vi "1CLABVIEW.vi"() -> ()   [LabVIEW 2013]
panel:
  out "CARRY":bool
  out "SUM":bool
  out "CARRY":bool
  out "SUM":bool
  in  "Cin":bool
  in  "B":bool
  in  "A":bool
  in  "B":bool
  in  "A":bool
  # "1(c).HALF ADDER and  FULL ADDER"
  # "O.SRINIVAS\n23A91A04H6"
  # "Half adder"
  # "Full adder"
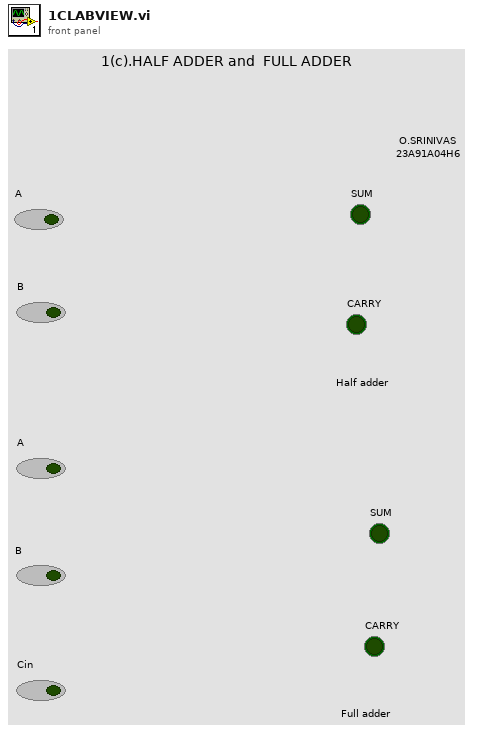
[diagram p1: front panel]
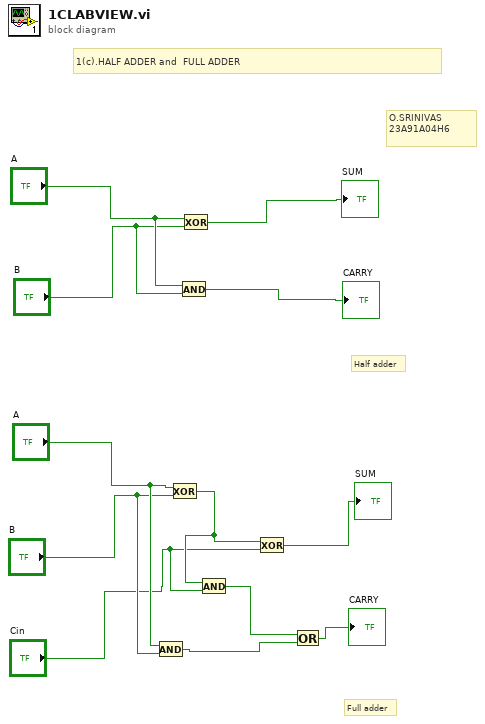
[diagram p0: block diagram]
diagram:
  # "Full adder"
  # "Half adder"
  # "1(c).HALF ADDER and  FULL ADDER"
  # "O.SRINIVAS\n23A91A04H6"
  n1 = And(x="A", y="B") -> (x .and. y?=w3:bool)
  n2 = Exclusive Or(1:"B", 2:"A") -> (0:w2:bool)
  n3 = And(x="A", y="B") -> (x .and. y?=→"CARRY":bool)
  n4 = Exclusive Or(1:"B", 2:"A") -> (0:→"SUM":bool)
  n5 = And(x=w2, y="Cin") -> (x .and. y?=w4:bool)
  n6 = Exclusive Or(1:"Cin", 2:w2) -> (0:→"SUM":bool)
  n7 = Or(x=w4, y=w3) -> (x .or. y?=→"CARRY":bool)
